vi "NF WF1973_74 OPC.vi"(6 "Read(F)":bool, 8 "error in (no error)":errorcluster caption="Error IN", 11 "VISAsession":refnum<visa-resource-name>) -> (0 "error out":errorcluster caption="Error OUT", 2 "Query OPC":i32=999, 3 "CopyVISAsession":refnum<visa-resource-name>)   [LabVIEW 2010]
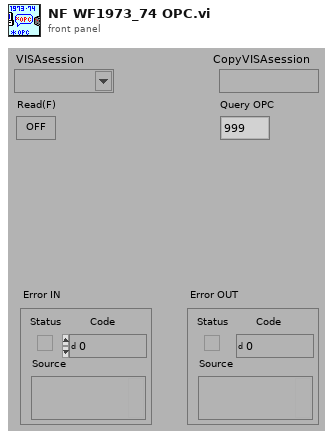
[diagram p1: front panel]
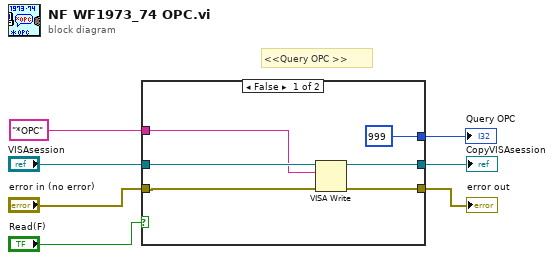
[diagram p0: block diagram]
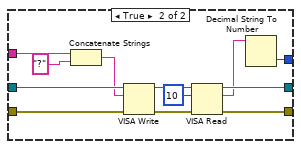
[diagram p2: hidden frame]
diagram:
  # "<<Query OPC >>"
  n1 = case shown="FALSE" "Read(F)" {
    tunnel: "VISAsession" -> [w10 w25]
    tunnel: [w12 w24] -> w6
    tunnel: [w13 w23] -> w5
    tunnel: "error in (no error)" -> [w11 w22]
    tunnel: "*OPC" ("文字列") -> [w9 w21]
    tunnel: [999 w20] -> w2
    frame False {
      n2 = VISA Write(VISA resource name=w10, write buffer=w9, error in (no error)=w11) -> (VISA resource name out=w12:refnum<visa-resource-name>, error out=w13:errorcluster)  [unwired: 1 out]
    }
    frame True {
      n3 = Concatenate Strings(w21, "?" ("形式文字列")) -> (w15:string)
      n4 = VISA Write(VISA resource name=w25, write buffer=w15, error in (no error)=w22) -> (VISA resource name out=w18:refnum<visa-resource-name>, error out=w19:errorcluster)  [unwired: 1 out]
      n5 = VISA Read(VISA resource name=w18, byte count=u32 10 ("バイトカウント（0）"), error in (no error)=w19) -> (VISA resource name out=w24:refnum<visa-resource-name>, read buffer=w14:string, error out=w23:errorcluster)  [unwired: 1 out]
      n6 = Decimal String To Number(string=w14) -> (number=w20:i32)  [unwired: 2 in, 1 out]
    }
  }
  "error out" <- w5
  "CopyVISAsession" <- w6
  "Query OPC" <- w2
